vi "Validate Instrument Addon Name.vi"(8 "Error In":errorcluster, 10 "Name In":string, 11 "Instrument Addon Refnum In":T1 format="%.0x") -> (0 "Error Out":errorcluster, 2 "Name Out":string, 3 "Instrument Addon Refnum Out":T1=18446744073709551615 format="%.0x")   [LabVIEW 2020, in "Instrument Addon Scripting API.lvlib"]
doc: "Verifies if the IA Name provided as an input parameter is not an empty string.\n\nInput: \nInstrument Addon Refnum In: represents the reference to the Instrument Addon Custom Device\nName In: represents the desired name for the Custom Device\n\nOutput:\nInstrument Addon Refnum Our: represents the reference to the Instrument Addon Custom Device provided as input\nName Out: represents the desired name provided as input"
uses:
  Instrument Addon Scripting API.lvlib
  <vilib>/NI VeriStand/Custom Device API/Custom Device Item Ref.ctl
  <vilib>/NI VeriStand/Custom Device API/Custom Device API.lvlib
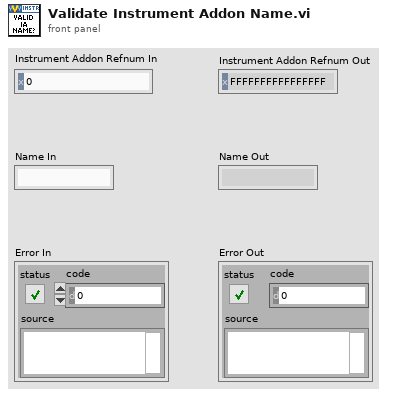
[diagram p1: front panel]
types:
  T1 = typedef "Custom Device API.lvlib/Custom Device Item Ref.ctl" = u64
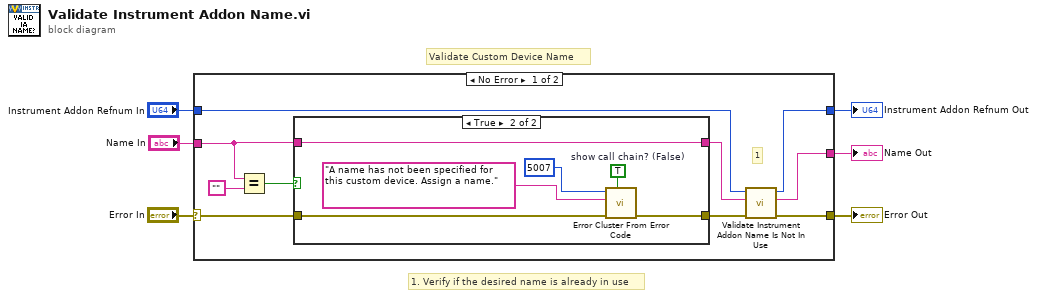
[diagram p0: block diagram]
diagram:
  # "1. Verify if the desired name is already in use"
  # "Validate Custom Device Name"
  n1 = case shown="No Error" "Error In" {
    selector: "Error In" -> [w14 w26]
    tunnel: "Name In" -> [w13 w27]
    tunnel: [w9 w25] -> w1
    tunnel: "Instrument Addon Refnum In" -> [w10 w25]
    tunnel: [w7 w26] -> w2
    tunnel: [w8 w27] -> w3
    frame No Error {
      # "1"
      n2 = Equal?(x=w13, y="") -> (x = y?=w15:bool)
      n3 = case shown="True" w15 {
        tunnel: w14 -> [w18 w21]
        tunnel: [w18 w23] -> w12
        tunnel: w13 -> [w17 w24]
        tunnel: [w17 w24] -> w11
        frame False {
        }
        frame True {
          w19 = TRUE  # show call chain? (False)
          n4 = call <vilib>:"Error Cluster From Error Code.vi"("show call chain? (False)"=w19, "error in (no error)"=w21, "error message (\"\")"="A name has not been specified for this custom device. Assign a name." ("error message (\"\")"), "error code (0)"=5007) -> ("error out"=w23:errorcluster)  [unwired: 5 in]
        }
      }
      n5 = call "Validate Instrument Addon Name Is Not In Use.vi"("Error In"=w12, "Name In"=w11, "Instrument Addon Refnum In"=w10) -> ("Error Out"=w7:errorcluster, "Name Out"=w8:string, "Instrument Addon Refnum Out"=w9:T1)  [unwired: 6 in]
    }
    frame Error {
    }
  }
  "Name Out" <- w3
  "Error Out" <- w2
  "Instrument Addon Refnum Out" <- w1
